vi "write servers jsons.vi"(8 "error in (no error)":errorcluster, 11 "Save Image in":refnum<class "Save Image.lvclass">) -> (0 "error out":errorcluster, 3 "Save Image out":refnum<class "Save Image.lvclass">)   [LabVIEW 2018, in "Save Image.lvclass"]
uses:
  Save Image.lvclass
  Save Image.lvclass/Save Image.ctl
  Channel/Channel.lvclass/Channel.ctl
  Header content/Header content.lvclass/Header content.ctl
  Server/Server.lvclass/Server.ctl
  State Machine/CCS_State Machine.lvclass
  RxTx/CCS_RxTx.lvclass
  Simulated_CCD_Camera/Simulated Camera.lvclass
  Header content/Header content.lvclass
  Log File/CCS_Log File.lvclass
  Error log/Error log.lvclass
  Keywords Log File/Keywords Log File.lvclass
  Server/Server.lvclass
  Channel/Channel.lvclass
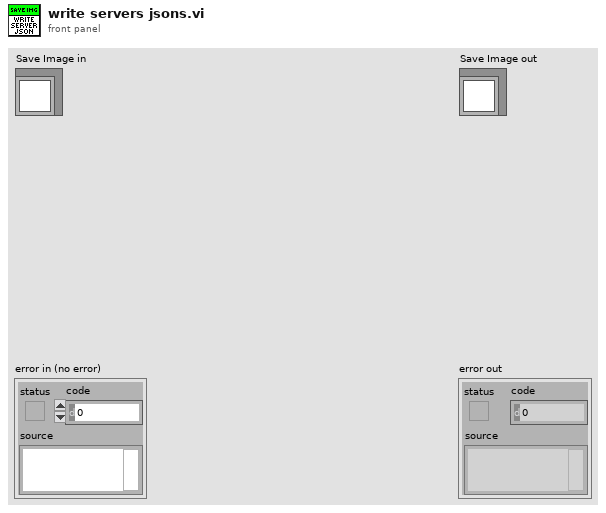
[diagram p1: front panel]
types:
  T1 = cluster{"State Machine.lvclass":refnum<class "CCS_State Machine.lvclass">, "RxTx.lvclass":refnum<class "CCS_RxTx.lvclass">, "Simulated_CCD_Camera.lvclass":refnum<class "Simulated Camera.lvclass">, "Save_Header_RxTx.lvclass":refnum<class "CCS_RxTx.lvclass">, "Header Content.lvclass":refnum<class "Header content.lvclass">, "Status SM.lvclass":refnum<class "CCS_State Machine.lvclass">, "Status RxTx.lvclass":refnum<class "CCS_RxTx.lvclass">, "Log File.lvclass":refnum<class "CCS_Log File.lvclass">, "Error log.lvclass":refnum<class "Error log.lvclass">, "Keywords Log File.lvclass":refnum<class "Keywords Log File.lvclass">}
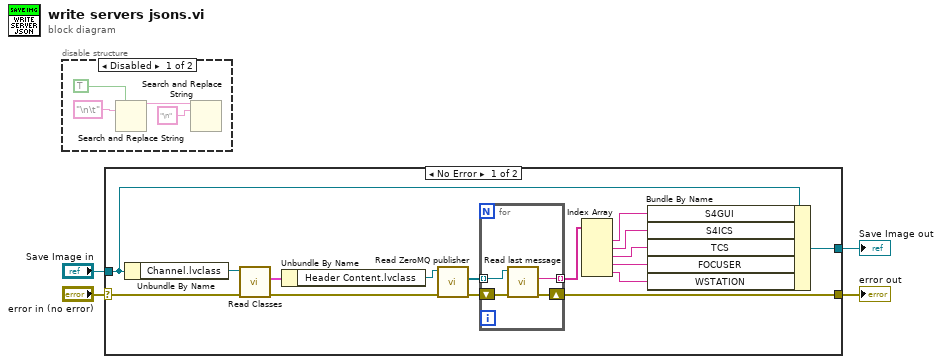
[diagram p0: block diagram]
diagram:
  n1 = disable-structure "Diagram Disable Structure" shown="Disabled" {
    frame Disabled {
      n2 = Search and Replace String(replace all?=TRUE ("replace all? (F)"), search string="\n\t") -> (result string=w8:string)  [unwired: 6 in, 3 out]
      n3 = Search and Replace String(input string=w8, search string="\n") -> ()  [unwired: 6 in, 4 out]
    }
    frame Enabled {
    }
  }
  n4 = case shown="No Error" "error in (no error)" {
    selector: "error in (no error)" -> [w19 w30]
    tunnel: [w17 w30] -> w3
    tunnel: [w15 w29] -> w1
    tunnel: "Save Image in" -> [w16 w29]
    frame No Error {
      n5 = Unbundle By Name(w16) -> ("Channel.lvclass"=w20:refnum<class "Channel.lvclass">)
      n6 = call "Read Classes.vi"("error in (no error)"=w19, "Channel in"=w20) -> ("error out"=w18:errorcluster, "Classes"=w21:T1)  [unwired: 7 in, 1 out]
      n7 = Unbundle By Name(w21) -> ("Header Content.lvclass"=w24:refnum<class "Header content.lvclass">)
      n8 = call "Read ZeroMQ publisher.vi"("error in (no error)"=w18, "Header content in"=w24) -> ("error out"=w22:errorcluster, "ZeroMQ publisher"=w23:refnum<class "Server.lvclass">[])  [unwired: 7 in, 1 out]
      n9 = for {
        tunnel: w23 -> [w28] mode=indexing
        tunnel: [w27] -> w14 mode=indexing
        shift-right: [w25] -> w17
        shift-left: w22 -> [w26]
        n10 = call "Read last message.vi"("error in (no error)"=w26, "Server in"=w28) -> ("error out"=w25:errorcluster, "last message"=w27:string)  [unwired: 7 in, 1 out]
      }
      n11 = Index Array(array=w14) -> (element #1=w13:string, element #2=w12:string, element #3=w11:string, element #4=w10:string, element #5=w9:string)  [unwired: 5 in]
      n12 = Bundle By Name(cluster=w16, "S4GUI"=w13, "S4ICS"=w12, "TCS"=w11, "FOCUSER"=w10, "WSTATION"=w9) -> (w15:refnum<class "Save Image.lvclass">)
    }
    frame Error {
    }
  }
  "error out" <- w3
  "Save Image out" <- w1
